vi "Teleop.vi"(10 "Match Info":T1={"Autonomous Elapsed Seconds"=0.0, "TeleOp Elapsed Seconds"=0.0, "Disabled Elapsed Seconds"=0.0, "Visited Autonomous"=FALSE, "Visited TeleOp"=FALSE, "Visited Disabled"=FALSE, "Autonomous Settings"={"Autonomous Style"=enum."Independent", "VI Refnum"=refnum}}, 11 "Call Context":T2) -> ()   [LabVIEW 2018]
doc: "This VI is called for each enabled TeleOp packet received from the DS. It is typically used to read from joysticks and other inputs and update I/O or setpoints for timed control loops. It should complete and return within 20 milliseconds or risk missing DS packets."
uses:
  <vilib>/Rock Robotics/WPI/DriverStation/WPI_DriverStationDerivedRobotMode.ctl
  <vilib>/Rock Robotics/WPI/DriverStation/WPI_DriverStationMatch Info.ctl
  <vilib>/Rock Robotics/WPI/Utilities/WPI_GetSetVariantRefNum.vi
  <vilib>/Rock Robotics/Network Tables/NT Write Boolean Array.vi
  <vilib>/Rock Robotics/Network Tables/NT Write Numeric Array.vi
  Framework/Robot Global Data.vi
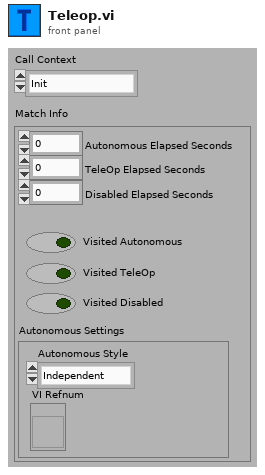
[diagram p1: front panel]
types:
  T1 = typedef "WPI_DriverStationMatch Info.ctl" = cluster{"Autonomous Elapsed Seconds":dbl, "TeleOp Elapsed Seconds":dbl, "Disabled Elapsed Seconds":dbl, "Visited Autonomous":bool, "Visited TeleOp":bool, "Visited Disabled":bool, "Autonomous Settings":cluster{"Autonomous Style":enum16{"Iterative", "Independent"}, "VI Refnum":refnum<vi>}}
  T2 = typedef "WPI_DriverStationDerivedRobotMode.ctl" = enum16{"Init", "Execute", "Stop"}
  T3 = typedef "WPI_JoystickDevRef.ctl" = cluster{"Device":T4}
  T4 = typedef "WPI_JoystickDeviceEnum.ctl" = enum16{"USB 0", "USB 1", "USB 2", "USB 3", "USB 4", "USB 5"}
  T5 = typedef "Command Status Info.ctl" = cluster{"Name":string, "Status":T6, "notifier out":T7}
  T6 = typedef "Completion Status.ctl" = enum16{"Successful", "Aborted", "Incomplete"}
  T7 = typedef "Completion Notifier.ctl" = refnum<notifier>
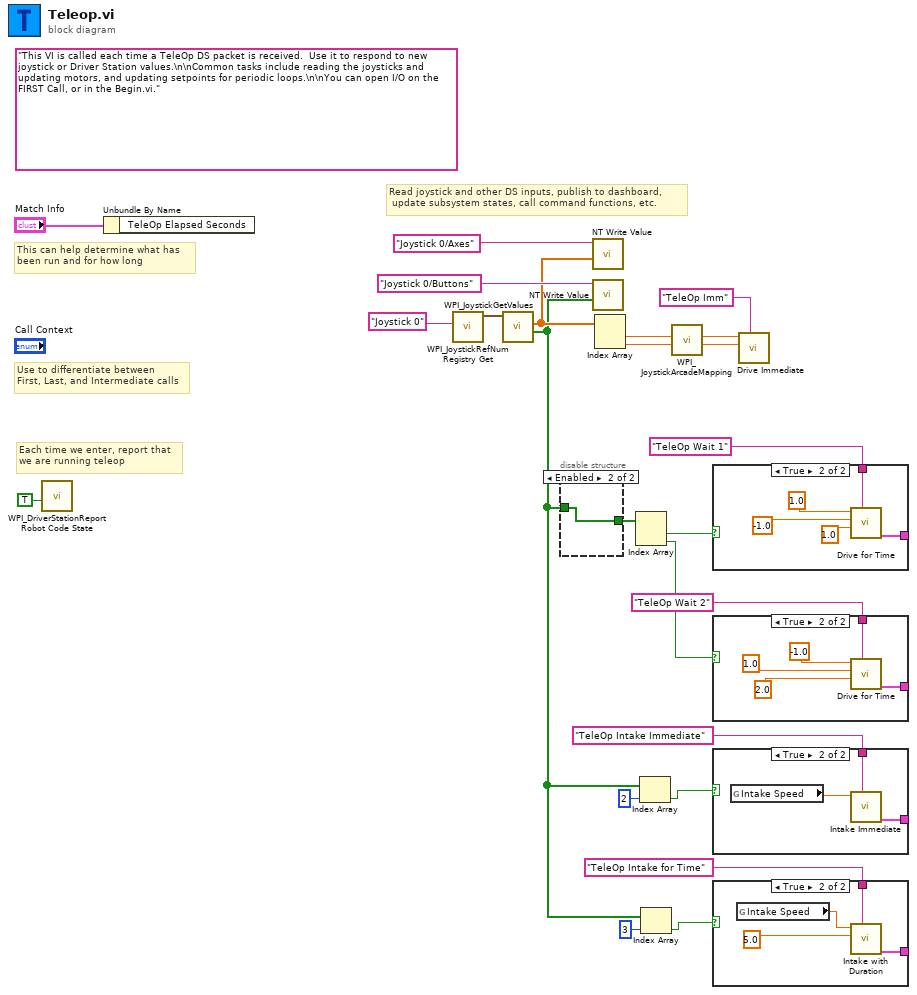
[diagram p0: block diagram]
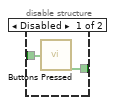
[diagram p4: hidden frame]
diagram:
  (unwired) "This VI is called each time a TeleOp DS packet is received.  Use it to respond to new joystick or Driver Station values.\n\nCommon tasks include reading the joysticks and updating motors, and updating setpoints for periodic loops.\n\nYou can open I/O on the FIRST Call, or in the Begin.vi."
  # "Read joystick and other DS inputs, publish to dashboard,\n update subsystem states, call command functions, etc."
  # "Each time we enter, report that\nwe are running teleop"
  # "Use to differentiate between\nFirst, Last, and Intermediate calls"
  # "This can help determine what has\nbeen run and for how long"
  n1 = call <vilib>:"WPI_DriverStationReport Robot Code State.vi"("TeleOp"=TRUE ("Autonomous")) -> ()  [unwired: 10 in, 1 out]
  n2 = Unbundle By Name("Match Info") -> ()  [unwired: 1 out]
  n3 = call <vilib>:"WPI_JoystickRefNum Registry Get.vi"("refnum name"="Joystick 0") -> ("JoystickDevRef"=w21:T3)  [unwired: 1 in, 9 out]
  n4 = call <vilib>:"WPI_JoystickGetValues.vi"("JoystickDevRef"=w21) -> ("Buttons"=w5:bool[], "Axes"=w9:dbl[])  [unwired: 6 in, 3 out]
  n5 = disable-structure shown="Enabled" {
    disable-tunnel: [w26 w27] -> w17
    disable-tunnel: w5 -> [w25 w27]
    frame Disabled {
      n6 = call "Buttons Pressed.vi"("Button Values"=w25) -> ("Button Presses"=w26:bool[])
    }
    frame Enabled {
    }
  }
  n7 = call-poly <vilib>:"NT Write Value.vi"("Numeric Array"=w9, "Name"="Joystick 0/Axes") -> ()  [unwired: 9 in, 1 out]
  n8 = call-poly <vilib>:"NT Write Value.vi"("Boolean Array"=w5, "Name"="Joystick 0/Buttons") -> ()  [unwired: 9 in, 1 out]
  n9 = Index Array(array=w9) -> (element #1=w12:dbl, element #2=w11:dbl)  [unwired: 2 in]
  n10 = Index Array(array=w17) -> (element #1=w16:bool, element #2=w15:bool)  [unwired: 2 in]
  n11 = Index Array(array=w5, index=2) -> (element=w4:bool)
  n12 = Index Array(array=w5, index=3) -> (element=w3:bool)
  n13 = call <vilib>:"WPI_JoystickArcadeMapping.vi"("Y axis value"=w11, "X axis value"=w12) -> ("Right Motor Value"=w13:dbl, "Left Motor Value"=w14:dbl)  [unwired: 8 in]
  n14 = case shown="True" w16 {
    tunnel: [_ w31] -> _
    tunnel: "TeleOp Wait 1" ("Description") -> [_ w30]
    frame False {
    }
    frame True {
      n15 = call "Drive for Time.vi"("Description"=w30, "Seconds"=1.0, "Right Speed"=-1.0, "Left Speed"=1.0) -> ("Command Info Out"=w31:T5)  [unwired: 7 in]
    }
  }
  n16 = case shown="True" w15 {
    tunnel: [_ w35] -> _
    tunnel: "TeleOp Wait 2" ("Description") -> [_ w34]
    frame False {
    }
    frame True {
      n17 = call "Drive for Time.vi"("Description"=w34, "Seconds"=2.0, "Right Speed"=1.0, "Left Speed"=-1.0) -> ("Command Info Out"=w35:T5)  [unwired: 7 in]
    }
  }
  n18 = case shown="True" w4 {
    tunnel: [_ w40] -> _
    tunnel: "TeleOp Intake Immediate" ("Description") -> [_ w39]
    frame False {
    }
    frame True {
      n19 = global read "Robot Global Data.vi" "Intake Speed"() -> (w38:dbl)
      n20 = call "Intake Immediate.vi"("Description"=w39, "Setpoint"=w38) -> ("Command Info Out"=w40:T5)  [unwired: 9 in]
    }
  }
  n21 = case shown="True" w3 {
    tunnel: [_ w44] -> _
    tunnel: "TeleOp Intake for Time" ("Description") -> [_ w43]
    frame False {
    }
    frame True {
      n22 = global read "Robot Global Data.vi" "Intake Speed"() -> (w41:dbl)
      n23 = call "Intake with Duration.vi"("Description"=w43, "Duration (s)"=5.0, "Setpoint"=w41) -> ("Command Info Out"=w44:T5)  [unwired: 8 in]
    }
  }
  n24 = call "Drive Immediate.vi"("Description"="TeleOp Imm", "Right Setpoint"=w13, "Left Setpoint"=w14) -> ()  [unwired: 8 in, 1 out]
